vi "Exercise 5.3 Webservice Webcam.vi"() -> ()   [LabVIEW 2014]
uses:
  <vilib>/Q-Wave Systems/QwaveSys RPi Training Package (Demo)/Addons/QwaveSys RPi Training Library.lvlib
  <vilib>/Q-Wave Systems/QwaveSys RPi Training Package (Demo)/Addons/WiringPi/WiringPi Pin Mode.ctl
  Desktop/.QwaveSys RPi Training Package/Exercises/Exercise 5 Webservice/temp.vi
  Desktop/.QwaveSys RPi Training Package/Exercises/Exercise 5 Webservice/led1.vi
  Desktop/.QwaveSys RPi Training Package/Exercises/Exercise 5 Webservice/led2.vi
  <vilib>/Q-Wave Systems/QwaveSys RPi Training Package (Demo)/Addons/WiringPi/WiringPi GPIO TypeDef.ctl
panel:
  out "GPIO5":bool
  out "GPIO1":bool
  out "Thermometer":dbl(slide) scale=15.0..40.0
  in  "file (use dialog)":path=path "/home/pi/temp.jpg"
  in  "webcamnum":i32
  in  "Image Size":T1(ring)
  in  "stop":bool
  out "Active":bool
  in  "LED2":T2=5 items=["Pin1_3.3V"=51, "Pin2_5V"=52, "Pin3_GPIO8_I2C1_SDA"=8, "Pin4_5V"=53, "Pin5_GPIO9_I2C1_SCL"=9, "Pin6_Gnd"=54, "Pin7_GPIO7_GPCLK0"=7, "Pin8_GPIO15_TXD_UART"=15, "Pin9_Gnd"=55, "Pin10_GPIO16_RXD_UART"=16, "Pin11_GPIO0"=0, "Pin12_GPIO1_PCMCLK_PWM0"=1, "Pin13_GPIO2"=2, "Pin14_Gnd"=56, "Pin15_GPIO3"=3, "Pin16_GPIO4"=4, "Pin17_3V"=57, "Pin18_GPIO5"=5, "Pin19_GPIO12_MOSI(SPI)"=12, "Pin20_Gnd"=58, "Pin21_GPIO13_MISO(SPI)"=13, "Pin22_GPIO6"=6, "Pin23_GPIO14_CLK(SPI)"=14, "Pin24_GPIO10_CE0_SPI"=10, "Pin25_Gnd"=59, "Pin26_GPIO11_CE1_SPI"=11, "Pin27_SDA0_I2C_EEPROM"=60, "Pin28_SCL0_I2C_EEPROM"=61, "Pin_29_GPIO21_GPCLK1"=21, "Pin30_Gnd"=62, "Pin31_GPIO22_GPCLK2"=22, "Pin32_GPIO26_PWM0"=26, "Pin33_GPIO23_PWM1"=23, "Pin34_Gnd"=63, "Pin35_GPIO24_PCMFS_PWM1"=24, "Pin36_GPIO27"=27, "Pin37_GPIO25"=25, "Pin38_GPIO28_PCM_DIN"=28, "Pin39_Gnd"=64, "Pin40_GPIO29_PCM_DOUT"=29]
  in  "LED1":T2=1 items=["Pin1_3.3V"=51, "Pin2_5V"=52, "Pin3_GPIO8_I2C1_SDA"=8, "Pin4_5V"=53, "Pin5_GPIO9_I2C1_SCL"=9, "Pin6_Gnd"=54, "Pin7_GPIO7_GPCLK0"=7, "Pin8_GPIO15_TXD_UART"=15, "Pin9_Gnd"=55, "Pin10_GPIO16_RXD_UART"=16, "Pin11_GPIO0"=0, "Pin12_GPIO1_PCMCLK_PWM0"=1, "Pin13_GPIO2"=2, "Pin14_Gnd"=56, "Pin15_GPIO3"=3, "Pin16_GPIO4"=4, "Pin17_3V"=57, "Pin18_GPIO5"=5, "Pin19_GPIO12_MOSI(SPI)"=12, "Pin20_Gnd"=58, "Pin21_GPIO13_MISO(SPI)"=13, "Pin22_GPIO6"=6, "Pin23_GPIO14_CLK(SPI)"=14, "Pin24_GPIO10_CE0_SPI"=10, "Pin25_Gnd"=59, "Pin26_GPIO11_CE1_SPI"=11, "Pin27_SDA0_I2C_EEPROM"=60, "Pin28_SCL0_I2C_EEPROM"=61, "Pin_29_GPIO21_GPCLK1"=21, "Pin30_Gnd"=62, "Pin31_GPIO22_GPCLK2"=22, "Pin32_GPIO26_PWM0"=26, "Pin33_GPIO23_PWM1"=23, "Pin34_Gnd"=63, "Pin35_GPIO24_PCMFS_PWM1"=24, "Pin36_GPIO27"=27, "Pin37_GPIO25"=25, "Pin38_GPIO28_PCM_DIN"=28, "Pin39_Gnd"=64, "Pin40_GPIO29_PCM_DOUT"=29]
  out "error out":errorcluster
  in  "error in (no error)":errorcluster
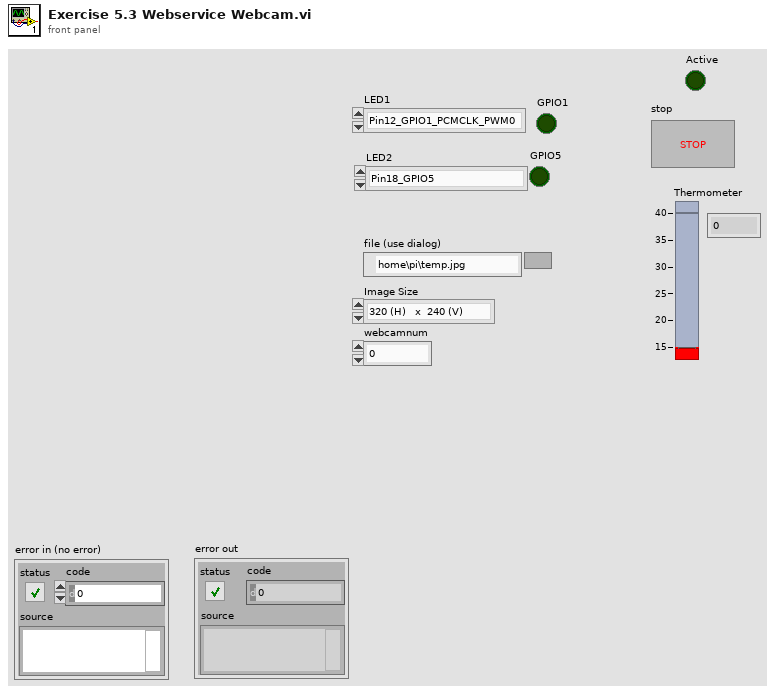
[diagram p1: front panel]
types:
  T1 = enum16{"320 (H)   x  240 (V)", "352(H)    x  288 (V)", "640 (H)   x  480 (V) ", "800 (H)   x  600 (V)", "1024 (H) x  768 (V)", "1280 (H) x  720 (V)", "1280 (H) x 1024 (V)", "1920 (H) x 1080 (V)"}
  T2 = typedef "QwaveSys RPi Training Library.lvlib/WiringPi GPIO TypeDef.ctl" = u8
  T3 = typedef "QwaveSys RPi Training Library.lvlib/WiringPi Pin Mode.ctl" = enum8{"INPUT", "OUTPUT", "PWM_OUTPUT", "GPIO_CLOCK", "SOFT_PWM_OUTPUT", "SOFT_TONE_OUTPUT", "PWM_TONE_OUTPUT"}
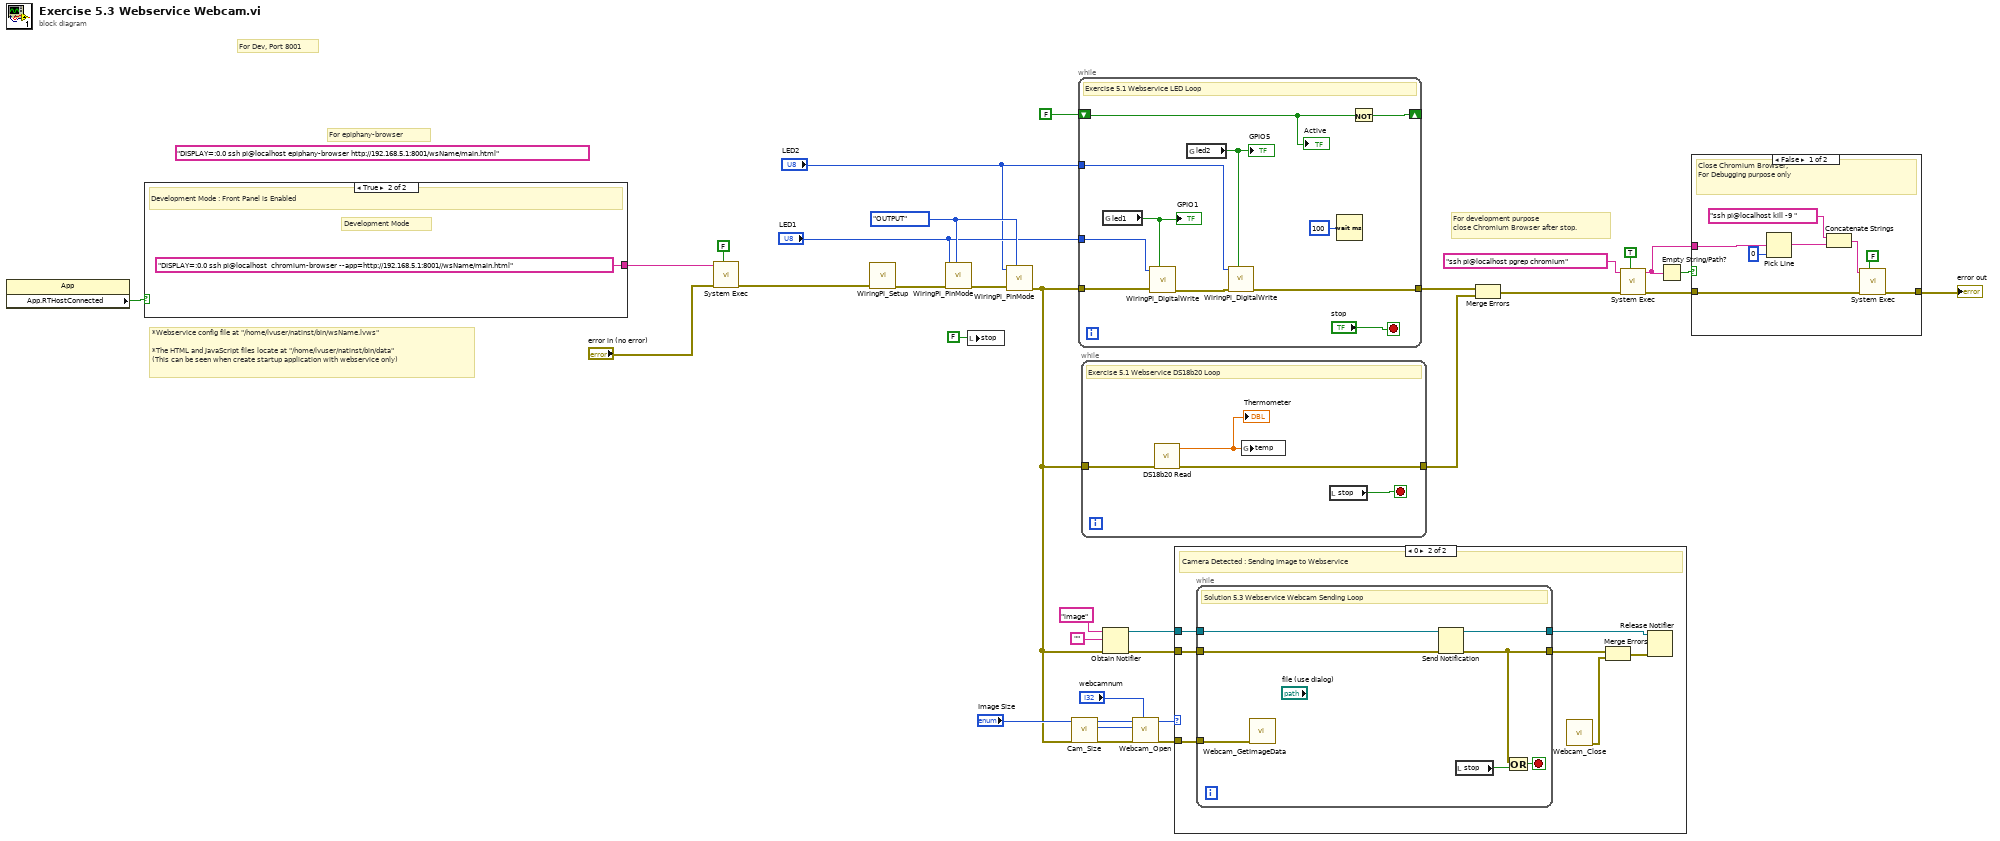
[diagram p0: block diagram]
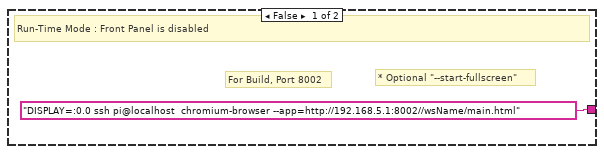
[diagram p3: hidden frame]
diagram:
  (unwired) "DISPLAY=:0.0 ssh pi@localhost epiphany-browser http://192.168.5.1:8001/wsName/main.html" ("command line")
  w31 = WiringPi_Pin_Mode."OUTPUT" ("Pin Mode")
  # "*Webservice config file at \"/home/lvuser/natinst/bin/wsName.lvws\"\n\n*The HTML and JavaScript files locate at \"/home/lvuser/natinst/bin/data\" \n(This can be seen when create startup application with webservice only)"
  # "For development purpose\nclose Chromium Browser after stop."
  # "For epiphany-browser"
  # "For Dev, Port 8001"
  n1 = property class="App"() -> ("App.RTHostConnected"=w13:bool)  [unwired: 2 in, 2 out]
  n2 = case shown="True" w13 {
    tunnel: ["DISPLAY=:0.0 ssh pi@localhost  chromium-browser --app=http://192.168.5.1:8002//wsName/main.html" ("command line") "DISPLAY=:0.0 ssh pi@localhost  chromium-browser --app=http://192.168.5.1:8001//wsName/main.html" ("command line")] -> w25
    frame False {
      # "For Build, Port 8002"
      # "* Optional \"--start-fullscreen\""
      # "Run-Time Mode : Front Panel is disabled"
    }
    frame True {
      # "Development Mode"
      # "Development Mode : Front Panel is Enabled"
    }
  }
  n3 = call <vilib>:"System Exec.vi"("wait until completion? (T)"=FALSE, "error in (no error)"="error in (no error)", "command line"=w25) -> ("error out"=w22:errorcluster)  [unwired: 5 in, 3 out]
  n4 = call <vilib>:"WiringPi_Setup.vi"("error in (no error)"=w22) -> ("error out"=w33:errorcluster)  [unwired: 10 in]
  n5 = call <vilib>:"WiringPi_PinMode.vi"("Pin Mode"=w31, "error in (no error)"=w33, "WiringPi GPIO"="LED1") -> ("error out"=w32:errorcluster)  [unwired: 8 in]
  n6 = local write "stop"(FALSE ("stop")) -> ()
  n7 = call <vilib>:"WiringPi_PinMode.vi"("Pin Mode"=w31, "error in (no error)"=w32, "WiringPi GPIO"="LED2") -> ("error out"=w2:errorcluster)  [unwired: 8 in]
  n8 = call <vilib>:"Cam_Size.vi"("error in (no error)"=w2, "Image Size"="Image Size") -> ("error out"=w7:errorcluster, "h"=w10:i32, "w"=w11:i32)  [unwired: 7 in]
  n9 = while {
    tunnel: w2 -> [w45]
    tunnel: "LED1" -> [w44]
    tunnel: "LED2" -> [w43]
    tunnel: [w42] -> w28
    shift-right: [w40] -> _
    shift-left: FALSE -> [w39]
    stop <- "stop" stop-if-true
    # "Exercise 5.1 Webservice LED Loop"
    n10 = global read "led1.vi" "led1"() -> (w37:bool)
    "GPIO1" <- w37
    n11 = call <vilib>:"WiringPi_DigitalWrite.vi"("Value"=w37, "error in (no error)"=w45, "WiringPi GPIO"=w44) -> ("error out"=w46:errorcluster)  [unwired: 8 in]
    n12 = global read "led2.vi" "led2"() -> (w36:bool)
    "GPIO5" <- w36
    n13 = call <vilib>:"WiringPi_DigitalWrite.vi"("Value"=w36, "error in (no error)"=w46, "WiringPi GPIO"=w43) -> ("error out"=w42:errorcluster)  [unwired: 8 in]
    n14 = Wait (ms)(milliseconds to wait=u32 100) -> ()  [unwired: 1 out]
    n15 = Not(x=w39) -> (.not. x?=w40:bool)
    "Active" <- w39
  }
  n16 = while {
    tunnel: w2 -> [w50]
    tunnel: [w49] -> w27
    stop <- w48 stop-if-true
    # "Exercise 5.1 Webservice DS18b20 Loop"
    n17 = call <vilib>:"DS18b20 Read.vi"("error in (no error)"=w50) -> ("error out"=w49:errorcluster, "Temp"=w47:dbl)  [unwired: 7 in, 2 out]
    "Thermometer" <- w47
    n18 = global write "temp.vi" "temp"(w47) -> ()
    n19 = local read "stop"() -> (w48:bool)
  }
  n20 = Obtain Notifier(name (unnamed)="image", notification data type="", error in (no error)=w2) -> (notifier out=w6:refnum<notifier>, error out=w4:errorcluster)  [unwired: 1 in, 1 out]
  n21 = call <vilib>:"Webcam_Open.vi"("webcamnum"="webcamnum", "error in (no error)"=w7, "height"=w10, "width"=w11) -> ("error out"=w8:errorcluster, "return type"=w1:i32)  [unwired: 6 in]
  n22 = case shown="0" w1 {
    tunnel: w8 -> [_ w57]
    tunnel: w6 -> [_ w56]
    tunnel: w4 -> [_ w55]
    frame -1, Default {
      # "NO Camera Found"
    }
    frame 0 {
      # "Camera Detected : Sending Image to Webservice"
      n23 = while {
        tunnel: w57 -> [w64]
        tunnel: w56 -> [w63]
        tunnel: w55 -> [w62]
        tunnel: [w60] -> w53
        tunnel: [w58] -> w51
        stop <- w59 stop-if-true
        # "Solution 5.3 Webservice Webcam Sending Loop"
        n24 = call <vilib>:"Webcam_GetImageData.vi"("error in (no error)"=w64) -> ()  [unwired: 8 in, 3 out]
        n25 = Send Notification(notifier=w63, error in (no error)=w62) -> (notifier out=w58:refnum<notifier>, error out=w60:errorcluster)  [unwired: 1 in]
        n26 = local read "stop"() -> (w61:bool)
        n27 = Or(x=w60, y=w61) -> (x .or. y?=w59:bool)
      }
      n28 = call <vilib>:"Webcam_Close.vi"() -> ("error out"=w52:errorcluster)  [unwired: 11 in]
      n29 = Merge Errors(w53, w52) -> (w54:errorcluster)
      n30 = Release Notifier(notifier=w51, error in (no error)=w54) -> ()  [unwired: 1 in, 3 out]
    }
  }
  n31 = Merge Errors(w28, w27) -> (w20:errorcluster)
  n32 = call <vilib>:"System Exec.vi"("wait until completion? (T)"=TRUE, "error in (no error)"=w20, "command line"="ssh pi@localhost pgrep chromium") -> ("error out"=w17:errorcluster, "standard output"=w16:string)  [unwired: 5 in, 2 out]
  n33 = Empty String/Path?(string/path=w16) -> (empty?=w18:bool)
  n34 = case shown="False" w18 {
    tunnel: w17 -> [w72 w73]
    tunnel: w16 -> [w71 _]
    tunnel: [w65 w73] -> w15
    frame False {
      # "Close Chromium Browser,\nFor Debugging purpose only"
      n35 = Pick Line(multi-line string=w71, line index=0) -> (output string=w68:string)  [unwired: 1 in]
      n36 = Concatenate Strings("ssh pi@localhost kill -9 " ("command line"), w68) -> (w67:string)
      n37 = call <vilib>:"System Exec.vi"("wait until completion? (T)"=FALSE, "error in (no error)"=w72, "command line"=w67) -> ("error out"=w65:errorcluster)  [unwired: 5 in, 3 out]
    }
    frame True {
      # "Chromium browser NOT running"
    }
  }
  "error out" <- w15
